vi "Configure Slit.vi"(7 "slit index (0)":u8, 8 "error in (no error)":errorcluster, 9 "reset (false)":bool, 10 "width, um":dbl, 11 "SOL MS in":refnum<class "PL SOL Instruments MS.lvclass">) -> (0 "error out":errorcluster, 2 "width, um":dbl, 3 "SOL MS out":refnum<class "PL SOL Instruments MS.lvclass">)   [LabVIEW 2015, in "PL SOL Instruments MS.lvclass"]
doc: "Configures slit."
uses:
  PL SOL Instruments MS.lvclass
  PL SOL Instruments MS.lvclass/PL SOL Instruments MS.ctl
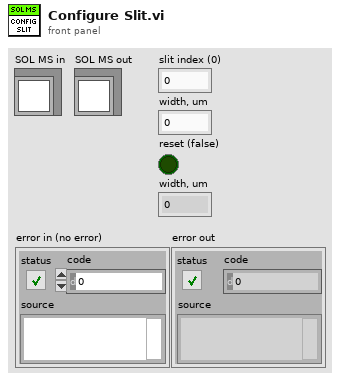
[diagram p1: front panel]
types:
  T1 = cluster{"name":string, "step timeout, ms":u32, "reset position":i32, "max position":i32, "backlash distance":i32, "step size, um":dbl, "current position":i32}[]
  T2 = cluster{"name":string, "step timeout, ms":u32, "reset position":i32, "max position":i32, "backlash distance":i32, "step size, um":dbl, "current position":i32}
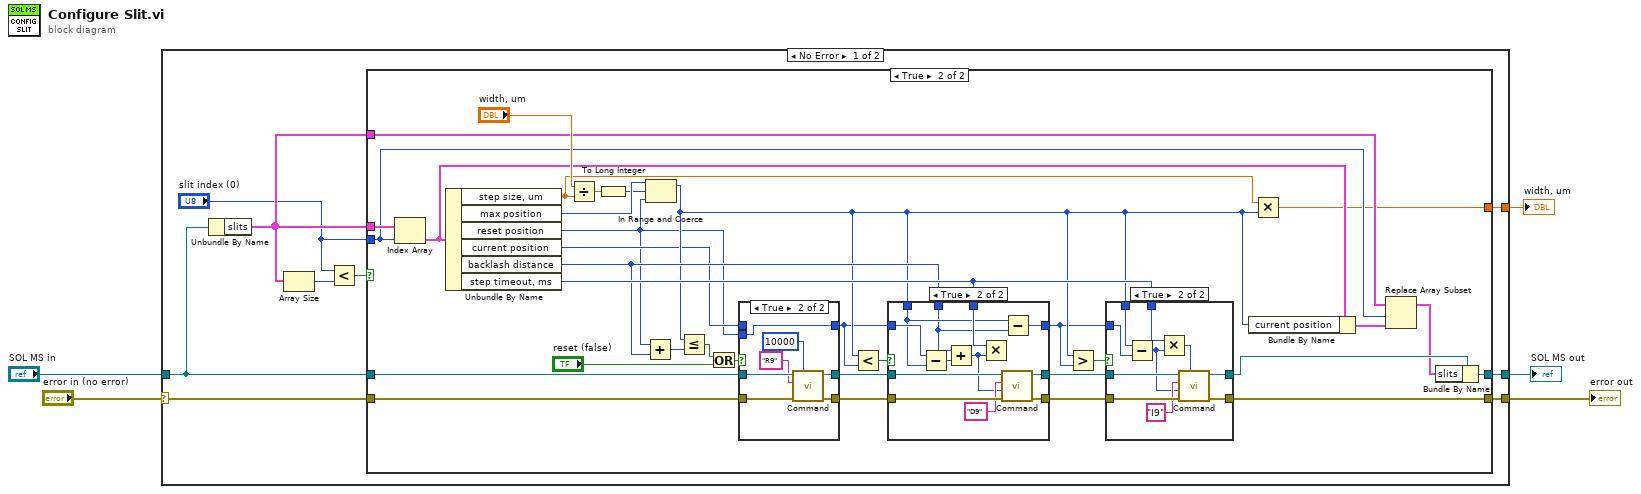
[diagram p0: block diagram]
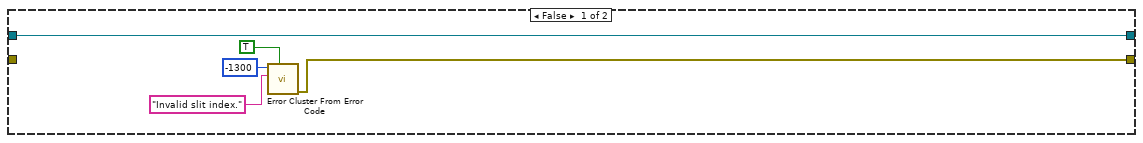
[diagram p2: hidden frame]
diagram:
  n1 = case shown="No Error" "error in (no error)" {
    selector: "error in (no error)" -> [w11 w91]
    tunnel: "SOL MS in" -> [w14 w92]
    tunnel: [w10 w92] -> w4
    tunnel: [w9 w91] -> w3
    tunnel: [w6 _] -> w1
    frame No Error {
      n2 = Unbundle By Name(w14) -> ("slits"=w8:T1)
      n3 = Array Size(array=w8) -> (size(s)=w13:i32)
      n4 = Less?(x="slit index (0)", y=w13) -> (x < y?=w12:bool)
      n5 = case shown="True" w12 {
        tunnel: w11 -> [_ w43]
        tunnel: w14 -> [w19 w44]
        tunnel: [w19 w37] -> w10
        tunnel: [w18 w36] -> w9
        tunnel: w8 -> [_ w53]
        tunnel: "slit index (0)" -> [_ w38]
        tunnel: w8 -> [_ w39]
        tunnel: [_ w34] -> w6
        frame False {
          n6 = call <vilib>:"Error Cluster From Error Code.vi"("show call chain? (False)"=TRUE, "error message (\"\")"="Invalid slit index." ("error message (\"\")"), "error code (0)"=-1300) -> ("error out"=w18:errorcluster)  [unwired: 6 in]
        }
        frame True {
          n7 = Index Array(array=w53, index=w38) -> (element=w40:T2)
          n8 = Unbundle By Name(w40) -> ("step size, um"=w35:dbl, "max position"=w47:i32, "reset position"=w48:i32, "current position"=w49:i32, "backlash distance"=w51:i32, "step timeout, ms"=w52:u32)
          n9 = Divide(x="width, um", y=w35) -> (x/y=w45:dbl)
          n10 = To Long Integer(number=w45) -> (32bit integer=w46:i32)
          n11 = Add(x=w48, y=w51) -> (x+y=w32:i32)
          n12 = In Range and Coerce(upper limit=w47, x=w46, lower limit=w48) -> (coerced(x)=w50:i32)  [unwired: 1 out]
          n13 = Less Or Equal?(x=w50, y=w32) -> (x <= y?=w31:bool)
          n14 = Or(x=w31, y="reset (false)") -> (x .or. y?=w33:bool)
          n15 = case shown="True" w33 {
            tunnel: w44 -> [w83 w89]
            tunnel: w43 -> [w82 w87]
            tunnel: [w82 w84] -> w28
            tunnel: [w83 w85] -> w29
            tunnel: w49 -> [w81 _]
            tunnel: [w81 w90] -> w27
            tunnel: w48 -> [_ w90]
            frame False {
            }
            frame True {
              n16 = call "Command.vi"("additional timeout, ms (0)"=u32 10000 ("timeout, ms (1000)"), "error in (no error)"=w87, "command"="R9", "SOL MS in"=w89) -> ("error out"=w84:errorcluster, "SOL MS out"=w85:refnum<class "PL SOL Instruments MS.lvclass">)  [unwired: 6 in]
            }
          }
          n17 = Less?(x=w50, y=w27) -> (x < y?=w30:bool)
          n18 = case shown="True" w30 {
            tunnel: w29 -> [w68 w74]
            tunnel: w28 -> [w67 w71]
            tunnel: [w67 w72] -> w26
            tunnel: [w68 w73] -> w25
            tunnel: w27 -> [w66 w78]
            tunnel: [w66 w77] -> w23
            tunnel: w50 -> [_ w76]
            tunnel: w51 -> [_ w75]
            tunnel: w52 -> [_ w79]
            frame False {
            }
            frame True {
              n19 = Subtract(x=w78, y=w76) -> (x-y=w80:i32)
              n20 = Add(x=w75, y=w80) -> (x+y=w69:i32)
              n21 = Multiply(x=w79, y=w69) -> ()  [unwired: 1 out]
              n22 = call "Command.vi"("error in (no error)"=w71, "data"=w69, "command"="D9", "SOL MS in"=w74) -> ("error out"=w72:errorcluster, "SOL MS out"=w73:refnum<class "PL SOL Instruments MS.lvclass">)  [unwired: 6 in]
              n23 = Subtract(x=w76, y=w75) -> (x-y=w77:i32)
            }
          }
          n24 = Greater?(x=w50, y=w23) -> (0:w24:bool)
          n25 = case shown="True" w24 {
            tunnel: w25 -> [w55 w62]
            tunnel: w26 -> [w54 w58]
            tunnel: [w54 w59] -> w36
            tunnel: [w55 w60] -> w22
            tunnel: w23 -> [_ w64]
            tunnel: w50 -> [_ w63]
            tunnel: w52 -> [_ w65]
            frame False {
            }
            frame True {
              n26 = Subtract(x=w63, y=w64) -> (x-y=w56:i32)
              n27 = Multiply(x=w65, y=w56) -> (x*y=w61:u32)
              n28 = call "Command.vi"("additional timeout, ms (0)"=w61, "error in (no error)"=w58, "data"=w56, "command"="I9", "SOL MS in"=w62) -> ("error out"=w59:errorcluster, "SOL MS out"=w60:refnum<class "PL SOL Instruments MS.lvclass">)  [unwired: 5 in]
            }
          }
          n29 = Bundle By Name(cluster=w40, "current position"=w50) -> (w21:T2)
          n30 = Multiply(x=w35, y=w50) -> (x*y=w34:dbl)
          n31 = Replace Array Subset(array=w39, new element=w21, index=w38) -> (w20:T1)
          n32 = Bundle By Name(cluster=w22, "slits"=w20) -> (w37:refnum<class "PL SOL Instruments MS.lvclass">)
        }
      }
    }
    frame Error {
    }
  }
  "SOL MS out" <- w4
  "error out" <- w3
  "width, um" <- w1
